vi "Send and Receive.vi"(6 "timeout (ms) [500]":i32, 8 "error in (no error)":errorcluster, 9 "Data":variant, 10 "Command":string, 11 "RemoteControl in":refnum<class "RemoteControl.lvclass">) -> (0 "error out":errorcluster, 1 "Data out":variant, 2 "Command out":string, 3 "RemoteControl out":refnum<class "RemoteControl.lvclass">)   [LabVIEW 2019, in "RemoteControl.lvlib" / "RemoteControl.lvclass"]
uses:
  RemoteControl.lvclass
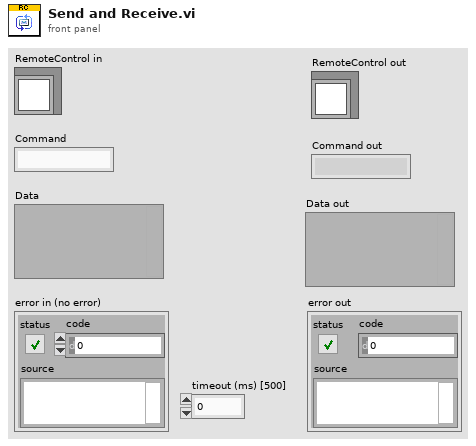
[diagram p1: front panel]
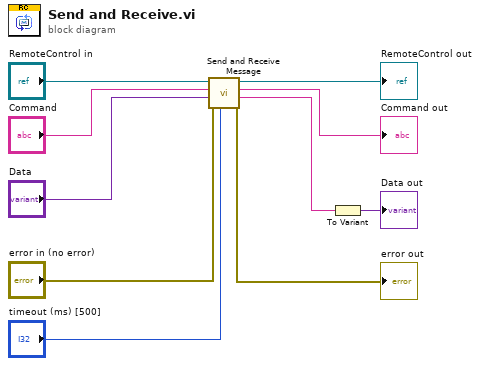
[diagram p0: block diagram]
diagram:
  n1 = call-dynamic "Send and Receive Message.vi"("timeout (ms) [500]"="timeout (ms) [500]", "error in (no error)"="error in (no error)", "Data"="Data", "Command"="Command", "RemoteControl in"="RemoteControl in") -> ("error out"=→"error out":errorcluster, "Data out"=w4:string, "Command out"=→"Command out":string, "RemoteControl out"=→"RemoteControl out":refnum<class "RemoteControl.lvclass">)  [unwired: 3 in]
  n2 = To Variant(anything=w4) -> (Variant=→"Data out":variant)
